vi "WriteConsumerState.vi"(8 "error in (no error)":errorcluster, 10 "Consumer State":string, 11 "Queue in":refnum<queue>) -> (0 "error out":errorcluster, 3 "Queue out":refnum<queue>)   [LabVIEW 2019]
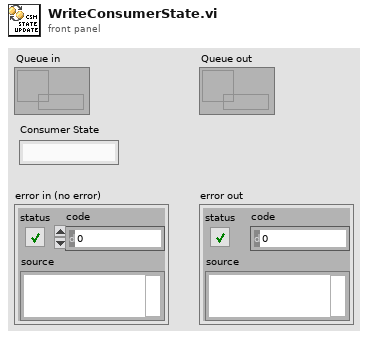
[diagram p1: front panel]
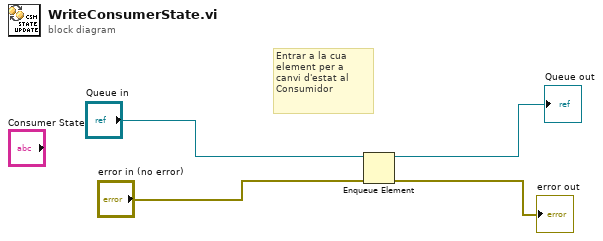
[diagram p0: block diagram]
diagram:
  # "Entrar a la cua element per a canvi d'estat al Consumidor"
  n1 = Enqueue Element(queue="Queue in", error in (no error)="error in (no error)") -> (queue out=→"Queue out":refnum<queue>, error out=→"error out":errorcluster)  [unwired: 2 in, 1 out]
